vi "Hollowness Score Finder.vi"(9 "Averages":dbl[](array[numeric]), 10 "Maximum":dbl[](array[numeric]), 11 "Minimum":dbl[](array[numeric])) -> (3 "Hollowness Score":dbl)   [LabVIEW 2013]
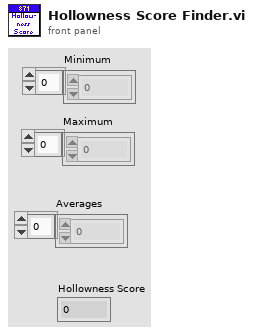
[diagram p1: front panel]
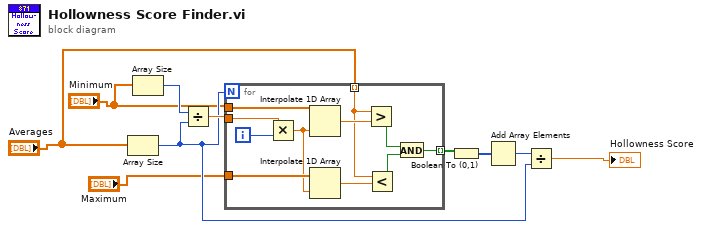
[diagram p0: block diagram]
diagram:
  n1 = Array Size(array="Averages") -> (size(s)=w5:i32)
  n2 = Array Size(array="Minimum") -> (size(s)=w9:i32)
  n3 = Divide(x=w9, y=w5) -> (x/y=w10:dbl)
  n4 = for {
    N: w5 -> [_]
    tunnel: w10 -> [w21]
    tunnel: "Minimum" -> [w19]
    tunnel: "Maximum" -> [w18]
    tunnel: "Averages" -> [w12] mode=indexing
    tunnel: [w11] -> w7 mode=indexing
    i -> [w20]
    n5 = Multiply(x=w21, y=w20) -> (x*y=w17:dbl)
    n6 = Interpolate 1D Array(1:w17, 2:w19) -> (0:w16:dbl)
    n7 = Interpolate 1D Array(1:w17, 2:w18) -> (0:w15:dbl)
    n8 = Greater?(x=w12, y=w16) -> (0:w14:bool)
    n9 = Less?(x=w12, y=w15) -> (x < y?=w13:bool)
    n10 = And(x=w14, y=w13) -> (x .and. y?=w11:bool)
  }
  n11 = Boolean To (0,1)(Boolean=w7) -> (0, 1=w8:i16[])
  n12 = Add Array Elements(numeric array=w8) -> (sum=w6:i16)
  n13 = Divide(x=w6, y=w5) -> (x/y=→"Hollowness Score":dbl)
